vi "INS_Driver_v1.10.vi"() -> ()   [LabVIEW 2017]
uses:
  IL Driver Library.lvlib
panel:
  out "error out":errorcluster
  in  "baud rate":T1(ring)
  in  "#COM Port":refnum<visa-resource-name>
  in  "?":bool
  in  "Stop read":bool
  in  "Start read":bool
  out "Cluster":T2 {"Altitude" format="%#_11g"; "Longitude" format="%#_11g"; "Latitude" format="%#_11g"}
  out "2D Picture":picture
  out "Gauge":i32(knob) scale=0.0..360.0
  out "QPVT":T3 {"Altitude" format="%#_11g"; "Longitude" format="%#_11g"; "Latitude" format="%#_11g"}
  out "Sensors":T4 {"Altitude" format="%#_11g"; "Longitude" format="%#_11g"; "Latitude" format="%#_11g"}
  out "Error":errorcluster
  in  "Error Window":bool caption="Cancel Button"
  in  "Output data format":T5(ring)
  in  "Accel range \n(g)":enum16{"2", "4", "6", "8", "10", "15", "40"}(ring)
  in  "Gyro rande \n(deg/sec)":T6(ring)
  # "Orientation angles (deg)"
  # "Sensors output"
  # "Rate(deg/s)"
  # "Accel(g)"
  # "Magn(nT)"
  # "X"
  # "Y"
  # "Z"
  # "Additional"
  # "Position abs (deg,m)"
  # "Quaternion of orientation"
  # "Sensors output"
  # "Rate(deg/s)"
  # "Accel(g)"
  # "Magn(nT)"
  # "X"
  # "Y"
  # "Z"
  # "Additional"
  # "Position abs (deg,m)"
  # "Orientation angles (deg)"
  # "Sensors output\n(ADC code)"
  # "Rate"
  # "Accel"
  # "Magn"
  # "X"
  # "Y"
  # "Z"
  # "Additional\n   (code)"
  # "Position abs (deg,m)"
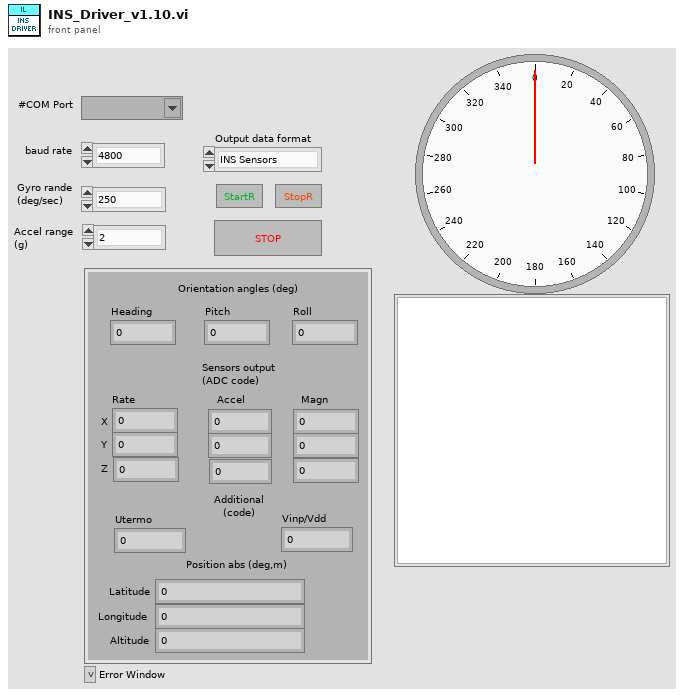
[diagram p1: front panel]
types:
  T1 = enum16{"4800", "9600", "14400", "19200", "38400", "57600", "115200", "230400", "460800", "921600"}
  T2 = cluster{"Heading":dbl, "Pitch":dbl, "Roll":dbl, "GyroX(deg/s)":dbl, "GyroY(deg/s)":dbl, "GyroZ(deg/s)":dbl, "AxelX(g)":dbl, "AxelY(g)":dbl, "AxelZ(g)":dbl, "Dec":i32, "MagY":i32, "MagZ":i32, "Temperature(deg C)":dbl, "Vinp(V)":dbl, "Latitude":dbl, "Longitude":dbl, "Altitude":dbl}
  T3 = cluster{"Lk0":dbl, "Lk1":dbl, "Lk2":dbl, "Lk3":dbl, "Numeric 5":dbl, "Numeric 6":dbl, "Numeric 7":dbl, "Numeric 8":dbl, "Numeric 9":dbl, "Numeric 10":dbl, i32, i32, i32, "Temperature(deg C)":dbl, "Vinp(V)":dbl, "Latitude":dbl, "Longitude":dbl, "Altitude":dbl}
  T4 = cluster{"Heading":dbl, "Pitch":dbl, "Roll":dbl, "GyroX(deg/s)":dbl, "GyroY(deg/s)":dbl, "GyroZ(deg/s)":dbl, "AxelX(g)":dbl, "AxelY(g)":dbl, "AxelZ(g)":dbl, "Dec":i32, "MagY":i32, "MagZ":i32, "Utermo":dbl, "Vinp/Vdd":dbl, "Latitude":dbl, "Longitude":dbl, "Altitude":dbl}
  T5 = enum16{"INS Sensors", "INS OPVT", "INS QPVT", "INS OPVT2A", "INS OPVT2AW", "INS OPVT2Ahr", "INS Minimal", "INS NMEA"}
  T6 = enum16{"250", "300", "450", "500", "1000", "2000"}
  T7 = cluster{string, string, string, string, string, string}
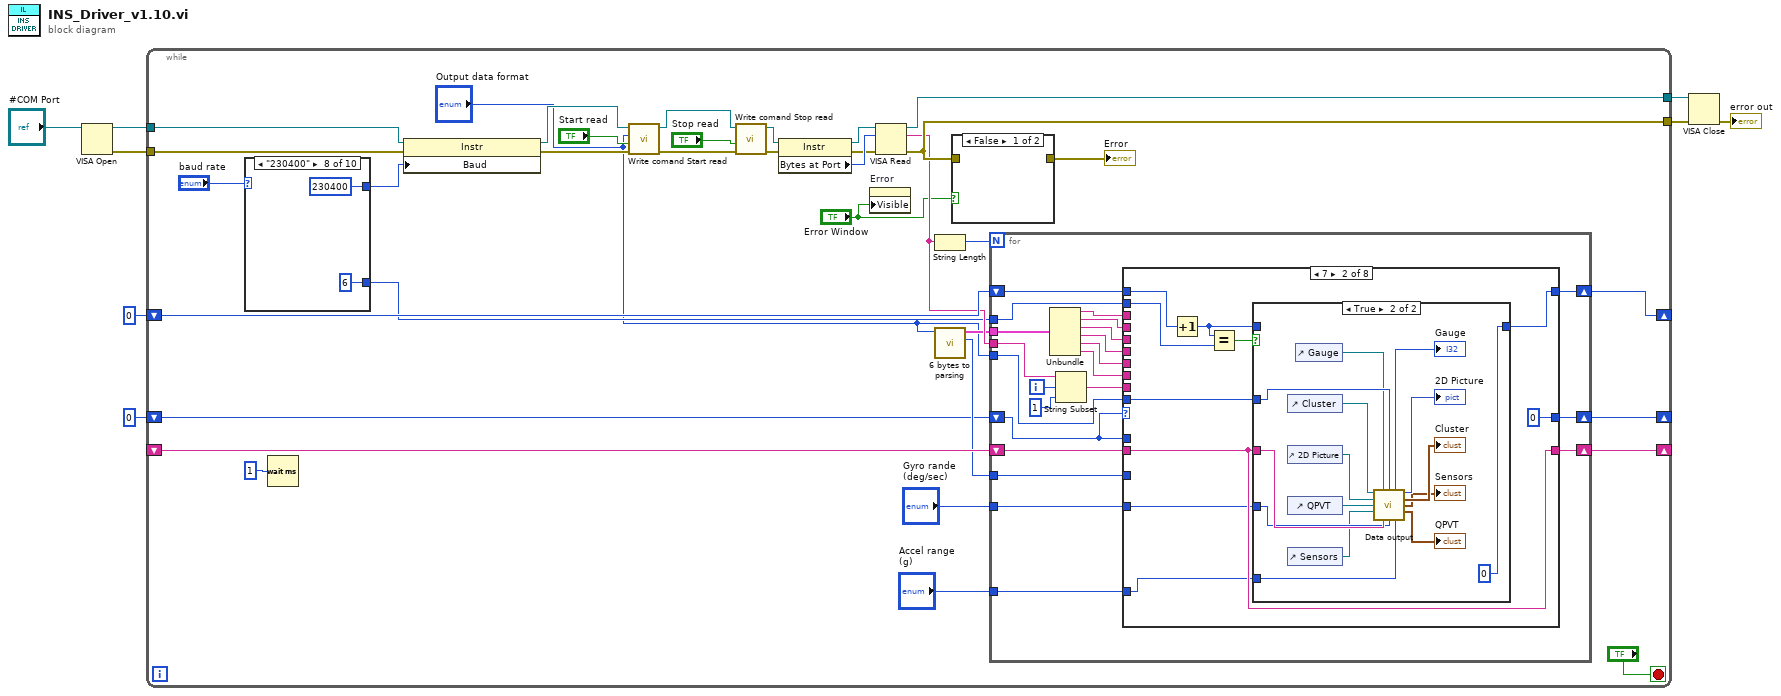
[diagram p0: block diagram]
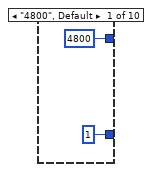
[diagram p3: hidden frame]
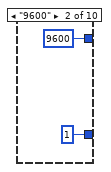
[diagram p4: hidden frame]
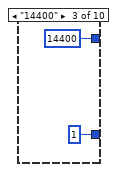
[diagram p5: hidden frame]
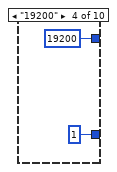
[diagram p6: hidden frame]
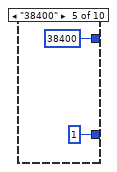
[diagram p7: hidden frame]
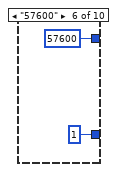
[diagram p8: hidden frame]
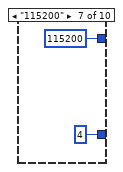
[diagram p9: hidden frame]
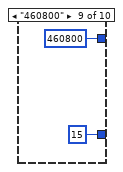
[diagram p10: hidden frame]
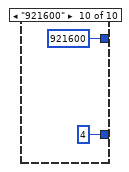
[diagram p11: hidden frame]
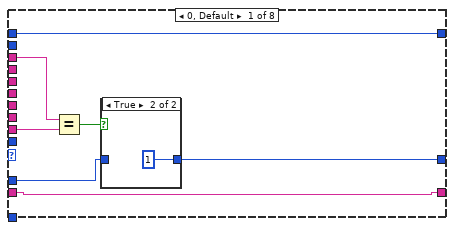
[diagram p12: hidden frame]
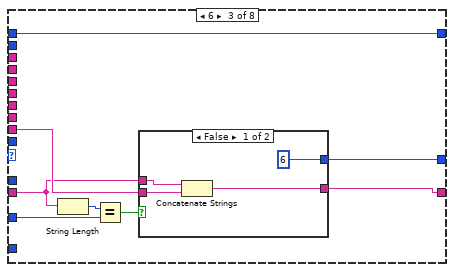
[diagram p15: hidden frame]
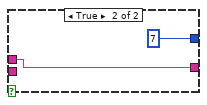
[diagram p16: hidden frame]
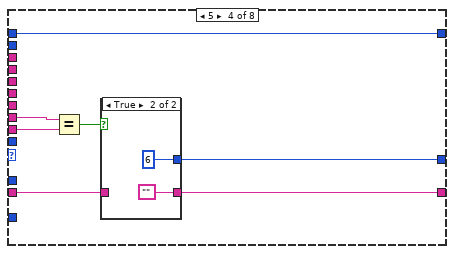
[diagram p17: hidden frame]
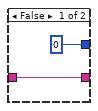
[diagram p18: hidden frame]
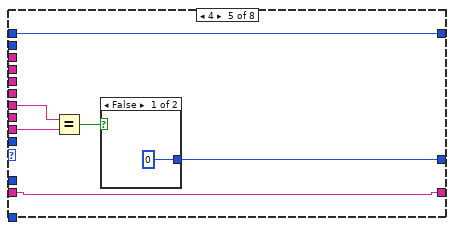
[diagram p19: hidden frame]
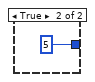
[diagram p20: hidden frame]
diagram:
  n1 = VISA Open(VISA resource name="#COM Port") -> (VISA resource name=w7:refnum<visa-resource-name>, error out=w8:errorcluster)  [unwired: 4 in]
  n2 = while {
    tunnel: w8 -> [w15]
    tunnel: w7 -> [w16]
    tunnel: [w39] -> w1
    tunnel: [w28] -> w3
    shift-right: [w30] -> _
    shift-left: _ -> [w32]
    shift-right: [w31] -> _
    shift-left: 0 -> [w23]
    shift-right: [w29] -> _
    shift-left: 0 -> [w25]
    stop <- "?" stop-if-true
    n3 = case shown="\"230400\"" "baud rate" {
      tunnel: [4800 9600 14400 19200 38400 57600 115200 230400 460800 921600] -> w17
      tunnel: [1 1 1 1 1 1 4 6 15 4] -> w18
      frame "4800", Default {
      }
      frame "9600" {
      }
      frame "14400" {
      }
      frame "19200" {
      }
      frame "38400" {
      }
      frame "57600" {
      }
      frame "115200" {
      }
      frame "230400" {
      }
      frame "460800" {
      }
      frame "921600" {
      }
    }
    n4 = Wait (ms)(milliseconds to wait=u32 1) -> ()  [unwired: 1 out]
    n5 = property class="Instr"(reference=w16, error in=w15, "Baud"=w17) -> (reference out=w14:refnum<visa-resource-name>, error out=w13:errorcluster)
    n6 = call "Write comand Start read.vi"("error in (no error)"=w13, "Start read"="Start read", "Output data format"="Output data format", "VISA Refnum in"=w14) -> ("error out"=w41:errorcluster, "VISA Refnum out"=w42:refnum<visa-resource-name>)  [unwired: 6 in]
    n7 = call "Write comand Stop read.vi"("error in (no error)"=w41, "Stop read"="Stop read", "VISA Refnum in"=w42) -> ("error out"=w36:errorcluster, "VISA Refnum out"=w37:refnum<visa-resource-name>)  [unwired: 7 in]
    n8 = property class="Instr"(reference=w37, error in=w36) -> (reference out=w33:refnum<visa-resource-name>, error out=w34:errorcluster, "Bytes at Port"=w35:u32)
    n9 = property on="Error" class="Clust (strict)"("Visible"="Error Window") -> ()  [unwired: 2 in, 2 out]
    n10 = VISA Read(VISA resource name=w33, byte count=w35, error in (no error)=w34) -> (VISA resource name out=w39:refnum<visa-resource-name>, read buffer=w24:string, error out=w28:errorcluster)  [unwired: 1 out]
    n11 = String Length(string=w24) -> (length=w38:i32)
    n12 = call "6 bytes to parsing.vi"("Output data format"="Output data format") -> ("data packet length"=w26:i32, "First 6 bytes"=w19:T7)  [unwired: 9 in]
    n13 = case shown="False" "Error Window" {
      tunnel: w28 -> [_ w44]
      tunnel: [_ w44] -> w10
      frame False {
      }
      frame True {
      }
    }
    "Error" <- w10
    n14 = for {
      N: w38 -> [_]
      tunnel: w24 -> [w86]
      shift-right: [w81] -> w30
      shift-left: w32 -> [w82]
      shift-right: [w77] -> w31
      shift-left: w23 -> [w78]
      shift-right: [w79] -> w29
      shift-left: w25 -> [w80]
      tunnel: w18 -> [w76]
      tunnel: w26 -> [w75]
      tunnel: "Output data format" -> [w74]
      tunnel: "Gyro rande \n(deg/sec)" -> [w73]
      tunnel: "Accel range \n(g)" -> [w72]
      tunnel: w19 -> [w71]
      i -> [w85]
      n15 = Unbundle(w71) -> (w70:string, w69:string, w68:string, w67:string, w66:string, w65:string)
      n16 = String Subset(string=w86, offset (0)=w85, length (rest)=1 ("length (rest)")) -> (substring=w83:string)
      n17 = case shown="7" w78 {
        tunnel: w83 -> [w93 _ w126 w141 w151 w159 w167 w176]
        tunnel: [w91 w103 w127 w139 w150 w158 w166 w174] -> w81
        tunnel: w82 -> [w91 w103 w125 w140 w150 w158 w166 w174]
        tunnel: w78 -> [w90 _ _ _ _ _ _ _]
        tunnel: w80 -> [w89 w105 w124 w138 w149 w157 w165 w173]
        tunnel: [w89 w104 w124 w138 w149 w157 w165 w173] -> w79
        tunnel: [w88 0 w123 w137 w148 w156 w164 w172] -> w77
        tunnel: w76 -> [_ w100 _ _ _ _ _ _]
        tunnel: w75 -> [_ _ w122 _ _ _ _ _]
        tunnel: w70 -> [w87 _ _ _ _ _ _ _]
        tunnel: w69 -> [_ _ _ _ _ _ _ w171]
        tunnel: w68 -> [_ _ _ _ _ _ w163 _]
        tunnel: w67 -> [_ _ _ _ _ w155 _ _]
        tunnel: w66 -> [_ _ _ _ w147 _ _ _]
        tunnel: w65 -> [_ _ _ w136 _ _ _ _]
        tunnel: w74 -> [_ w99 _ _ _ _ _ _]
        tunnel: w73 -> [_ w98 _ _ _ _ _ _]
        tunnel: w72 -> [_ w97 _ _ _ _ _ _]
        frame 0, Default {
          n18 = Equal?(x=w87, y=w93) -> (x = y?=w92:bool)
          n19 = case shown="True" w92 {
            tunnel: w90 -> [w94 _]
            tunnel: [w94 1] -> w88
            frame False {
            }
            frame True {
            }
          }
        }
        frame 7 {
          n20 = Increment(x=w105) -> (x+1=w101:i32)
          n21 = Equal?(x=w101, y=w100) -> (x = y?=w102:bool)
          n22 = case shown="True" w102 {
            tunnel: w103 -> [_ w119]
            tunnel: [w106 0] -> w104
            tunnel: w101 -> [w106 _]
            tunnel: w99 -> [_ w120]
            tunnel: w98 -> [_ w118]
            tunnel: w97 -> [_ w117]
            frame False {
            }
            frame True {
              n23 = control-ref of="Cluster"() -> (w116:refnum<vi>)
              n24 = control-ref of="2D Picture"() -> (w114:refnum<vi>)
              n25 = control-ref of="QPVT"() -> (w113:refnum<vi>)
              n26 = control-ref of="Sensors"() -> (w112:refnum<vi>)
              n27 = control-ref of="Gauge"() -> (w115:refnum<vi>)
              n28 = call "Data output .vi"("Cluster in"=w116, "Knob Refnum"=w115, "Output data format"=w120, "Pict Refnum"=w114, "Clust Refnum in"=w113, "Clust Refnum 3"=w112, "String"=w119, "Gyro rande \n(deg/sec)"=w118, "Accel range \n(g)"=w117) -> ("Gauge"=→"Gauge":i32, "2D Picture"=→"2D Picture":picture, "Cluster"=→"Cluster":T2, "Sensors"=→"Sensors":T4, "QPVT"=→"QPVT":T3)  [unwired: 2 in]
            }
          }
        }
        frame 6 {
          n29 = String Length(string=w125) -> (length=w129:i32)
          n30 = Equal?(x=w129, y=w122) -> (x = y?=w128:bool)
          n31 = case shown="False" w128 {
            tunnel: w125 -> [w133 w135]
            tunnel: w126 -> [w132 _]
            tunnel: [w131 w135] -> w127
            tunnel: [6 7] -> w123
            frame False {
              n32 = Concatenate Strings(w133, w132) -> (w131:string)
            }
            frame True {
            }
          }
        }
        frame 5 {
          n33 = Equal?(x=w136, y=w141) -> (x = y?=w142:bool)
          n34 = case shown="True" w142 {
            tunnel: [w144 ""] -> w139
            tunnel: w140 -> [w144 _]
            tunnel: [0 6] -> w137
            frame False {
            }
            frame True {
            }
          }
        }
        frame 4 {
          n35 = Equal?(x=w147, y=w151) -> (x = y?=w152:bool)
          n36 = case shown="False" w152 {
            tunnel: [0 5] -> w148
            frame False {
            }
            frame True {
            }
          }
        }
        frame 3 {
          n37 = Equal?(x=w155, y=w159) -> (x = y?=w160:bool)
          n38 = case shown="False" w160 {
            tunnel: [0 4] -> w156
            frame False {
            }
            frame True {
            }
          }
        }
        frame 2 {
          n39 = Equal?(x=w163, y=w167) -> (x = y?=w168:bool)
          n40 = case shown="True" w168 {
            tunnel: [0 3] -> w164
            frame False {
            }
            frame True {
            }
          }
        }
        frame 1 {
          n41 = Equal?(x=w171, y=w176) -> (x = y?=w175:bool)
          n42 = case shown="True" w175 {
            tunnel: [0 2] -> w172
            frame False {
            }
            frame True {
            }
          }
        }
      }
    }
  }
  n43 = VISA Close(VISA resource name=w1, error in (no error)=w3) -> (error out=→"error out":errorcluster)
